vi "TSCAN_GetSignalValue.vi"(4 "ALLSignalName":string[][](array[string]), 6 "ALLMessage":string[](array[string]), 7 "ALLID":i32[](array[numeric]) format="%x", 8 "簇":T1, 11 "路径输入":path) -> (0 "数组":string[](array[string]), 1 "元素索引":i32, 2 "SigValue":dbl[](array[numeric]), 3 "路径输出":path)   [LabVIEW 2019]
panel:
  out "tsdb_load_can_db":i32
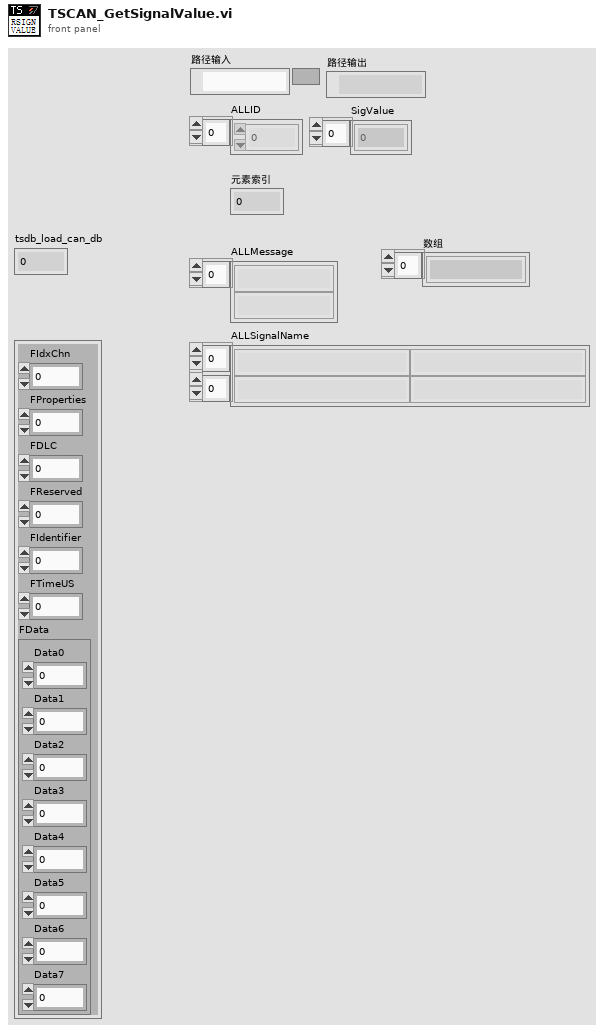
[diagram p1: front panel]
types:
  T1 = cluster{"FIdxChn":u8, "FProperties":u8, "FDLC":u8, "FReserved":u8, "FIdentifier":i32, "FTimeUS":u64, "FData":cluster{"Data0":u8, "Data1":u8, "Data2":u8, "Data3":u8, "Data4":u8, "Data5":u8, "Data6":u8, "Data7":u8}}
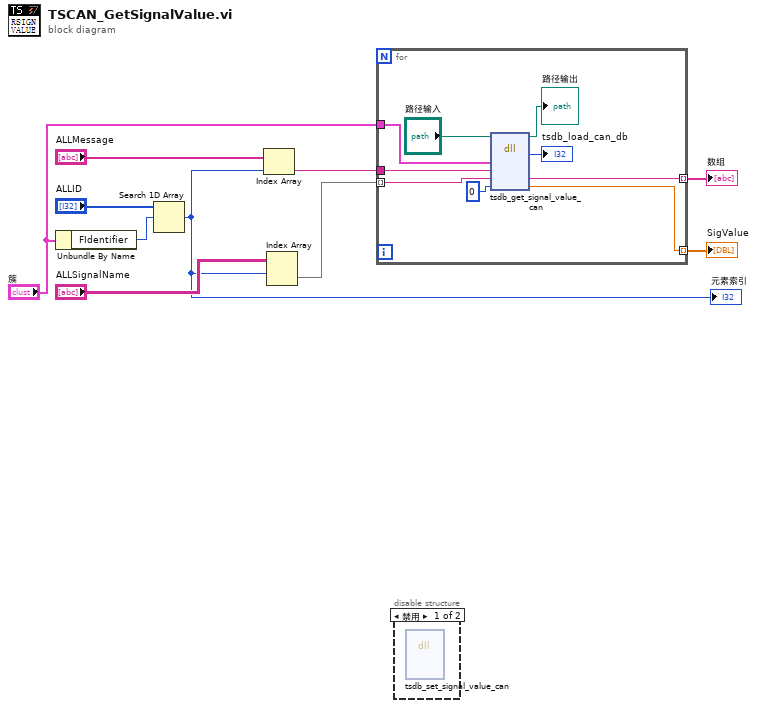
[diagram p0: block diagram]
diagram:
  n1 = Unbundle By Name("簇") -> ("FIdentifier"=w8:i32)
  n2 = Search 1D Array(1D array="ALLID", element=w8) -> (index of element=w4:i32)  [unwired: 1 in]
  "元素索引" <- w4
  n3 = Index Array(array="ALLMessage", index=w4) -> (element=w6:string)
  n4 = Index Array(array="ALLSignalName", index (row)=w4) -> (element=w3:string[])  [unwired: 1 in]
  n5 = for {
    tunnel: "簇" -> [w19]
    tunnel: w6 -> [w18]
    tunnel: w3 -> [w13] mode=indexing
    tunnel: [w12] -> w2 mode=indexing
    tunnel: [w11] -> w1 mode=indexing
    n6 = dll-call lib="PTH27abs EDemo同星\nTSCAN_V1.0ConfigTSMaster.dll" fn="tsdb_get_signal_value_can"(path in="路径输入", "CANObJ"=w19, "Message"=w18, "Signal"=w13, "SigValue"=0) -> (path out=→"路径输出":path, "tsdb_get_signal_value_can"=→"tsdb_load_can_db":i32, "Signal"=w11:string, "SigValue"=w12:dbl)  [unwired: 4 in, 1 out]
  }
  "SigValue" <- w2
  "数组" <- w1
  n7 = disable-structure shown="禁用" {
    frame Disabled {
      n8 = dll-call lib="PTH27abs EDemo同星\nTSCAN_V1.0ConfigTSMaster.dll" fn="tsdb_set_signal_value_can"() -> ()  [unwired: 10 in, 2 out]
    }
    frame Enabled {
    }
  }
